vi "signalgen.vi"() -> ()   [LabVIEW 2013]
uses:
  <vilib>/Analysis/1siggen.llb/Ramp Pattern by Samples.vi
  <vilib>/Analysis/NI_AALBase.lvlib
panel:
  out "error out":errorcluster
  out "VISA resource name out":refnum<visa-resource-name>
  in  "VISA resource name 3":refnum<visa-resource-name>
  in  "error in (no error) 3":errorcluster
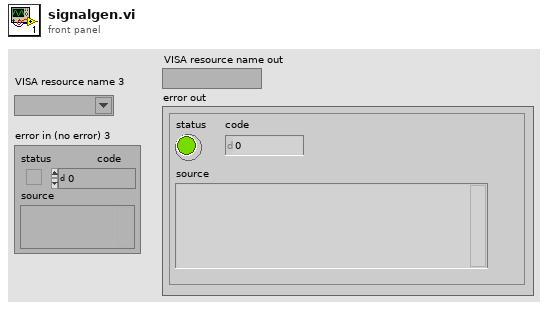
[diagram p1: front panel]
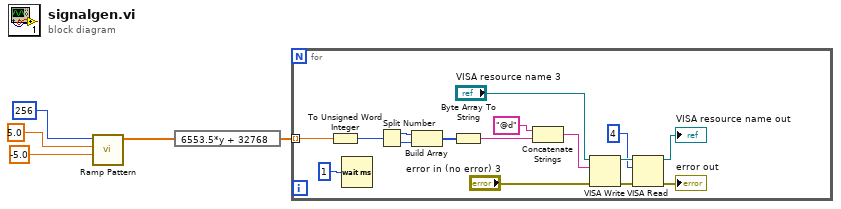
[diagram p0: block diagram]
diagram:
  n1 = call-poly <vilib>:"Ramp Pattern.vi"("start"=-5.0, "end"=5.0, "samples"=256) -> ("Ramp Pattern"=w1:dbl[])  [unwired: 7 in, 1 out]
  n2 = expression code="6553.5*y + 32768"(w1) -> (w3:dbl[])
  n3 = for {
    tunnel: w3 -> [w6] mode=indexing
    n4 = To Unsigned Word Integer(number=w6) -> (unsigned 16bit integer=w20:u16)
    n5 = Wait (ms)(milliseconds to wait=u32 1) -> ()  [unwired: 1 out]
    n6 = Split Number(x=w20) -> (hi(x)=w17:u8, lo(x)=w18:u8)
    n7 = Build Array(w17, w18) -> (w21:u8[])
    n8 = Byte Array To String(unsigned byte array=w21) -> (string=w19:string)
    n9 = Concatenate Strings("@d" ("write buffer"), w19) -> (w11:string)
    n10 = VISA Write(VISA resource name="VISA resource name 3", write buffer=w11, error in (no error)="error in (no error) 3") -> (VISA resource name out=w13:refnum<visa-resource-name>, error out=w14:errorcluster)  [unwired: 1 out]
    n11 = VISA Read(VISA resource name=w13, byte count=u32 4, error in (no error)=w14) -> (VISA resource name out=→"VISA resource name out":refnum<visa-resource-name>, error out=→"error out":errorcluster)  [unwired: 2 out]
  }
